vi "UART Read.vi"() -> ()   [LabVIEW 2020, in "CTI-Scratchpad.lvlib"]
uses:
  CTI-Scratchpad.lvlib
  CTI/UART Number.ctl
  CTI/GPIO Number.ctl
  CTI/Session/Session.lvclass
  CTI/VisaComms/VisaComms.lvclass
  CTI/CTI.lvlib
panel:
  out "String":string
  in  "stop":bool
  in  "RX GPIO":T1=17
  in  "TX GPIO":T1=16
  in  "Baud":u32=9600
  in  "UART":T2=1
  in  "Port":refnum<visa-resource-name>="COM5"
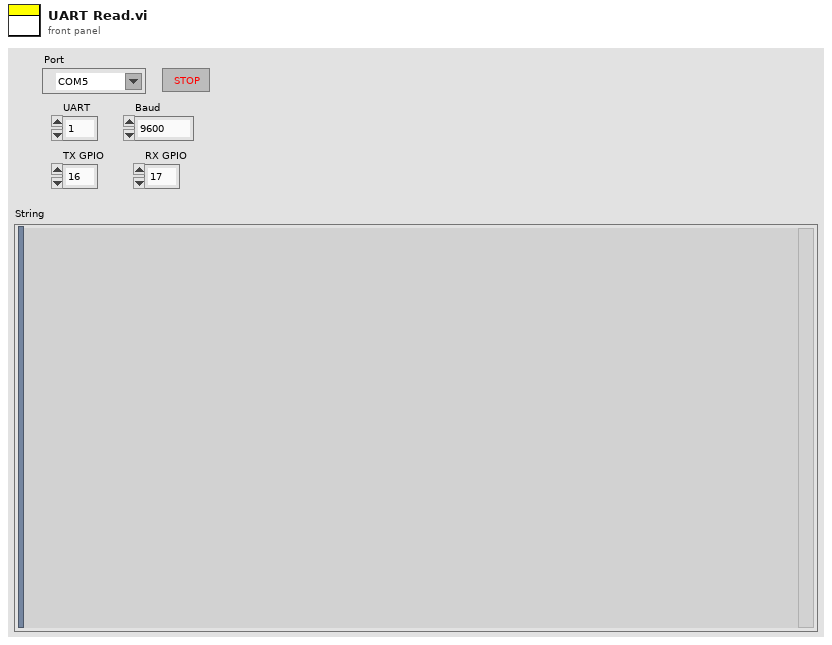
[diagram p1: front panel]
types:
  T1 = typedef "CTI.lvlib/GPIO Number.ctl" = i8
  T2 = typedef "CTI.lvlib/UART Number.ctl" = i8
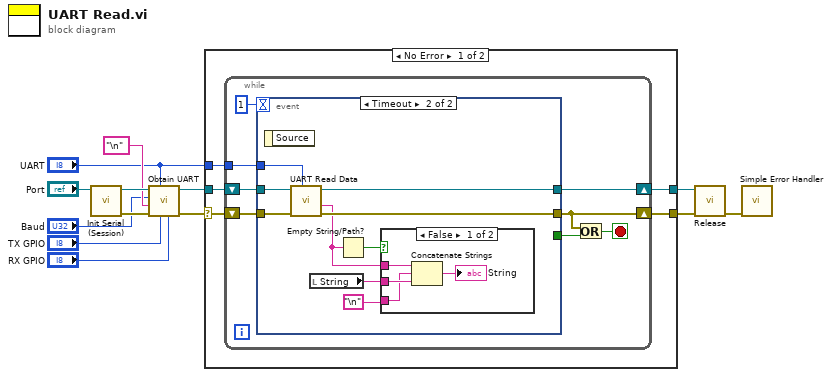
[diagram p0: block diagram]
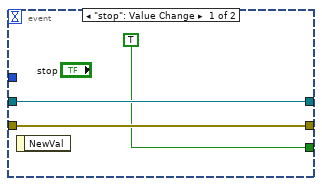
[diagram p2: hidden frame]
diagram:
  n1 = call "Init Serial (Session).vi"("VISA resource name in"="Port") -> ("error out"=w11:errorcluster, "Session"=w12:refnum<class "Session.lvclass">)  [unwired: 8 in, 1 out]
  n2 = call "Obtain UART.vi"("RX GPIO"="RX GPIO", "TX GPIO"="TX GPIO", "UART #"="UART", "error in (no error)"=w11, "Term Char (None)"="\n", "Baud"="Baud", "Session in"=w12) -> ("error out"=w10:errorcluster, "Session out"=w9:refnum<class "Session.lvclass">)  [unwired: 3 in]
  n3 = case shown="No Error" w10 {
    selector: w10 -> [w16 w44]
    tunnel: w9 -> [w17 w43]
    tunnel: "UART" -> [w18 _]
    tunnel: [w15 w44] -> w8
    tunnel: [w14 w43] -> w7
    frame No Error {
      n4 = while {
        tunnel: w18 -> [w25]
        shift-right: [w24] -> w14
        shift-left: w17 -> [w26]
        shift-right: [w22] -> w15
        shift-left: w16 -> [w23]
        stop <- w20 stop-if-true
        n5 = event shown="[1] Timeout" {
          selector: _ -> [_ _]
          dyn-events: _ -> [_ _]
          timeout: 1 -> [_ _]
          tunnel: w26 -> [w29 w38]
          tunnel: w25 -> [_ w30]
          tunnel: [w29 w35] -> w24
          tunnel: w23 -> [w28 w37]
          tunnel: [w28 w36] -> w22
          tunnel: [TRUE _] -> w21
          event "stop": Value Change {
            n6 = event-data() -> ()  [unwired: 1 in, 1 out]
          }
          event Timeout {
            n7 = event-data() -> ()  [unwired: 1 in, 1 out]
            n8 = call "UART Read Data.vi"("UART #"=w30, "error in (no error)"=w37, "Session in"=w38) -> ("error out"=w36:errorcluster, "Data"=w31:string, "Session out"=w35:refnum<class "Session.lvclass">)  [unwired: 6 in]
            n9 = local read "String"() -> (w34:string)
            n10 = Empty String/Path?(string/path=w31) -> (empty?=w33:bool)
            n11 = case shown="False" w33 {
              tunnel: w34 -> [w42 _]
              tunnel: w31 -> [w41 _]
              tunnel: "\n" -> [w39 _]
              frame False {
                n12 = Concatenate Strings(w41, w39, w42) -> (→"String":string)
              }
              frame True {
              }
            }
          }
        }
        n13 = Or(x=w22, y=w21) -> (x .or. y?=w20:bool)
      }
    }
    frame Error {
    }
  }
  n14 = call-dynamic "Release.vi"("error in (no error)"=w8, "Session in"=w7) -> ("error out"=w6:errorcluster)  [unwired: 9 in]
  n15 = call <vilib>:"Simple Error Handler.vi"("error in (no error)"=w6) -> ()  [unwired: 4 in, 5 out]
